vi "Set Engine Simulation Toolkit Custom Device.vi"(8 "error in (no error)":errorcluster, 10 "Settings":T1 {"Rate decimation" min=1}, 11 "EST Custom Device in":refnum<k24>) -> (0 "error out":errorcluster, 3 "EST Custom Device out":refnum<k24>)   [LabVIEW 2015, in "Engine Simulation Toolkit Scripting API.lvlib"]
uses:
  Engine Simulation Toolkit Scripting API.lvlib
  Engine Simulation Toolkit Custom Device Settings.ctl
  NationalInstruments.VeriStand.SystemDefinitionAPI
  Shared/Properties.vi
  <vilib>/NI Veristand/Custom Device API/Set Item Property (I32).vi
  <vilib>/NI VeriStand/Custom Device API/Custom Device API.lvlib
  Shared/Engine Simulation Toolkit Shared.lvlib
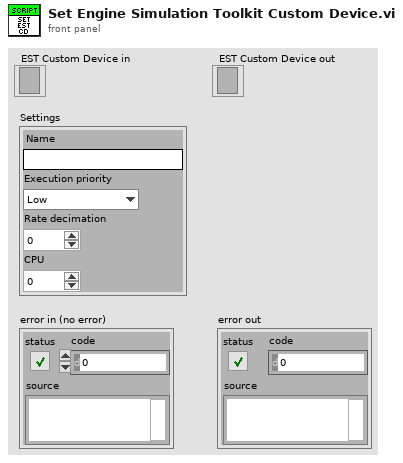
[diagram p1: front panel]
types:
  T1 = typedef "Engine Simulation Toolkit Scripting API.lvlib/Engine Simulation Toolkit Custom Device Settings.ctl" = cluster{"Name":string, "Execution priority":enum16{"Low", "Medium", "High"}, "Rate decimation":i32, "CPU":i32}
  T2 = typedef "Custom Device API.lvlib/Custom Device Item Ref.ctl" = u64
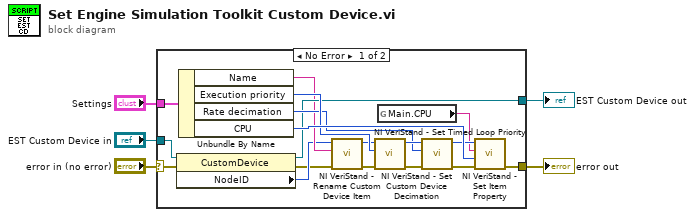
[diagram p0: block diagram]
diagram:
  n1 = case shown="No Error" "error in (no error)" {
    selector: "error in (no error)" -> [w12 w25]
    tunnel: "Settings" -> [w23 _]
    tunnel: [w22 w25] -> w4
    tunnel: [w13 w24] -> w3
    tunnel: "EST Custom Device in" -> [w11 w24]
    frame No Error {
      n2 = property class="CustomDevice"(reference=w11, error in=w12) -> (reference out=w13:refnum<k24>, error out=w6:errorcluster, "NodeID"=w9:u64)
      n3 = Unbundle By Name(w23) -> ("Name"=w10:string, "Execution priority"=w16:enum16{"Low", "Medium", "High"}, "Rate decimation"=w14:i32, "CPU"=w19:i32)
      n4 = call <vilib>:"NI VeriStand - Rename Custom Device Item.vi"("error in (no error)"=w6, "New Name"=w10, "Item Ref in"=w9) -> ("error out"=w7:errorcluster, "Item Ref out"=w8:T2)  [unwired: 6 in, 1 out]
      n5 = call <vilib>:"NI VeriStand - Set Timed Loop Priority.vi"("error in (no error)"=w7, "Priority"=w16, "Device Ref in"=w8) -> ("error out"=w21:errorcluster, "Device Ref out"=w15:T2)  [unwired: 7 in]
      n6 = global read "Properties.vi" "Main.CPU"() -> (w17:string)
      n7 = call <vilib>:"NI VeriStand - Set Custom Device Decimation.vi"("error in (no error)"=w21, "Decimation"=w14, "Device Ref in"=w15) -> ("error out"=w20:errorcluster, "Device Ref out"=w18:T2)  [unwired: 7 in]
      n8 = call-poly <vilib>:"NI VeriStand - Set Item Property.vi"("error in (no error)"=w20, "Value"=w19, "Property Name"=w17, "Item Ref in"=w18) -> ("error out"=w22:errorcluster)  [unwired: 5 in, 2 out]
    }
    frame Error {
    }
  }
  "error out" <- w4
  "EST Custom Device out" <- w3
